vi "FPGA Inverse Time Delay.vi"   [LabVIEW 2012, in "NI_EP_Protection_FPGA.lvlib"]
doc: "Delays for the time interval that you specify in the Inverse Time Curves VI before the trip signal asserts. The Inverse Time Curves VI generates inverse time curves for this VI to use. You can compensate for the processing delay of the input energizing quantity under a specific G/Gs in the Inverse Time Curves VI to achieve higher operate time accuracy."
uses:
  <vilib>/addons/Electrical Power/Protection/NI_EP_Protection_FPGA.lvlib
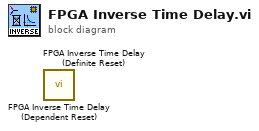
[diagram p0: block diagram]
diagram:
  n1 = call <vilib>:"FPGA Inverse Time Delay (Dependent Reset).vi"() -> ()  [unwired: 12 in, 4 out]
  n2 = call <vilib>:"FPGA Inverse Time Delay (Definite Reset).vi"() -> ()  [unwired: 12 in, 4 out]
